vi "Read Buffer.vi"(8 "error in (no error)":errorcluster, 11 "VISA resource name":refnum<visa-resource-name>) -> (0 "error out":errorcluster, 1 "Buffer Metadata":T1(array[cluster]), 2 "Buffer":dbl[](array[numeric]), 3 "VISA resource name out":refnum<visa-resource-name>)   [LabVIEW 2011, in "Keithley 2182.lvlib"]
doc: "Reads the contents of the buffer.\n\n<B>Note:</B>\nBuffer must first be enabled and configured using <Enable Buffer Storage</B> and <B>Configure Buffer</B> VIs."
uses:
  Keithley 2182.lvlib
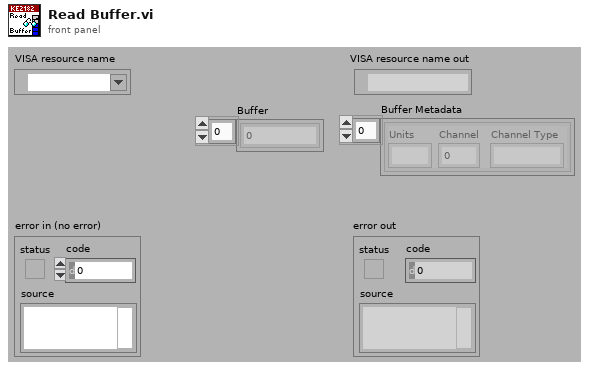
[diagram p1: front panel]
types:
  T1 = cluster{"Units":string, "Channel":i32, "Channel Type":string}[]
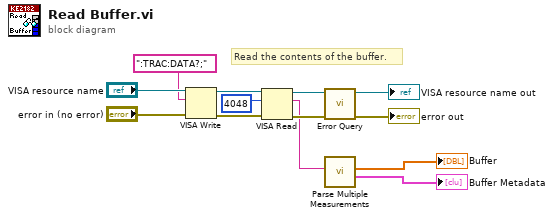
[diagram p0: block diagram]
diagram:
  # "Read the contents of the buffer."
  n1 = VISA Write(VISA resource name="VISA resource name", write buffer=":TRAC:DATA?;", error in (no error)="error in (no error)") -> (VISA resource name out=w7:refnum<visa-resource-name>, error out=w8:errorcluster)  [unwired: 1 out]
  n2 = VISA Read(VISA resource name=w7, byte count=u32 4048, error in (no error)=w8) -> (VISA resource name out=w4:refnum<visa-resource-name>, read buffer=w3:string, error out=w5:errorcluster)  [unwired: 1 out]
  n3 = call "Error Query.vi"("error in (no error)"=w5, "VISA resource name"=w4) -> ("error out"=→"error out":errorcluster, "VISA resource name out"=→"VISA resource name out":refnum<visa-resource-name>)  [unwired: 6 in, 2 out]
  n4 = call "Parse Multiple Measurements.vi"("Measurement String"=w3) -> ("Measurements Metadata"=→"Buffer Metadata":T1, "Measurements"=→"Buffer":dbl[])  [unwired: 9 in]
